vi "Set StimulationPK.vi"(8 "error in (no error)":errorcluster, 10 "StimulationPK":T1, 11 "BehaviorData in":refnum<class "BehaviorData.lvclass">) -> (0 "error out":errorcluster, 3 "BehaviorData out":refnum<class "BehaviorData.lvclass">)   [LabVIEW 2011, in "BehaviorData.lvclass"]
uses:
  BehaviorData.lvclass
  Database/StimulationPrimary.ctl
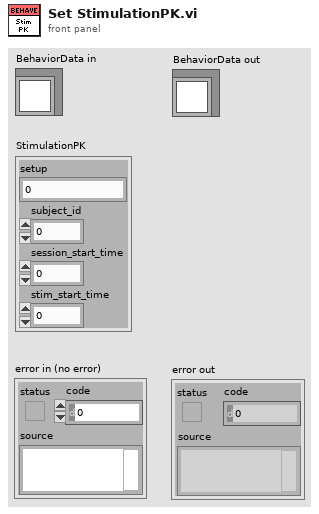
[diagram p1: front panel]
types:
  T1 = typedef "StimulationPrimary.ctl" = cluster{"setup":u8, "subject_id":i32, "session_start_time":dbl, "stim_start_time":dbl}
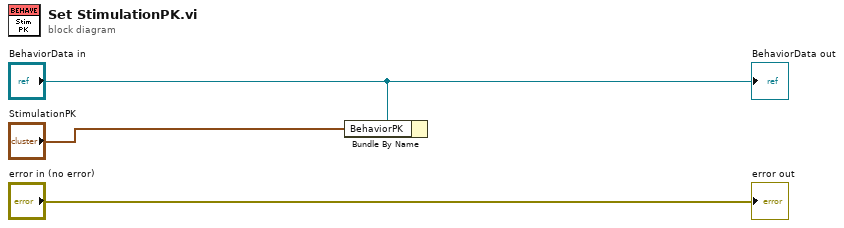
[diagram p0: block diagram]
diagram:
  n1 = Bundle By Name(cluster="BehaviorData in", "BehaviorPK"="StimulationPK") -> ()  [unwired: 1 out]
  "error out" <- "error in (no error)"
  "BehaviorData out" <- "BehaviorData in"
